vi "CRYdB ref to dB-ref string.vi"(6 "base prefix/unit":string, 7 "dB ref":dbl format="%.2f") -> (3 "dB/ref string":string)   [LabVIEW 2013]
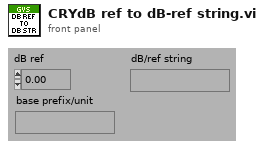
[diagram p1: front panel]
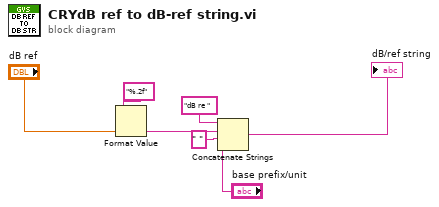
[diagram p0: block diagram]
diagram:
  n1 = Format Value(format string="%.2f", value (0)="dB ref") -> (output string=w4:string)  [unwired: 1 in]
  n2 = Concatenate Strings("dB re " ("format string"), w4, " " ("output string"), "base prefix/unit") -> (→"dB/ref string":string)
